vi "Example.vi"() -> ()   [LabVIEW 2014, in "DAQ HVPS.lvclass"]
uses:
  Session Based/DAQ/DAQ HVPS.lvclass
  Session Based/Base/Session HVPS.lvclass
  <userlib>/_Session Fwk/Session - Root.lvclass
  reusable/Session APIs/File Access/Config Data/Config Data.lvclass
  reusable/Session APIs/File Access/Config Data/Config Session.ctl
panel:
  in  "V 2":dbl
  out "x-y":u32
  out "error out":errorcluster
  out "V":dbl
  in  "Boolean":bool
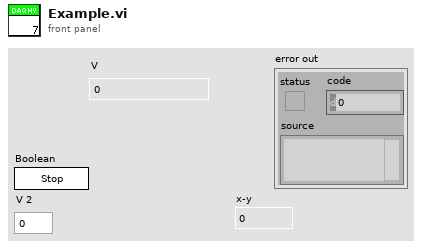
[diagram p1: front panel]
types:
  T1 = typedef "Config Data.lvclass/Config Session.ctl" = refnum<data-value>
  T2 = typedef "Session - Root.lvclass/Session Handle.ctl" = refnum<data-value>
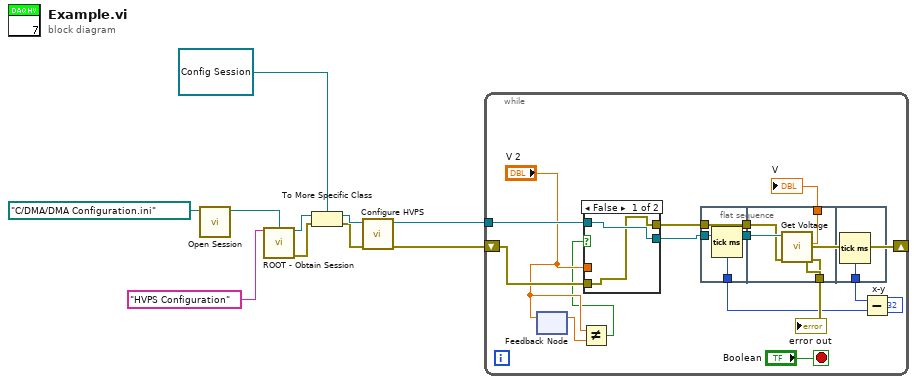
[diagram p0: block diagram]
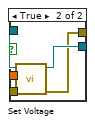
[diagram p2: hidden frame]
diagram:
  n1 = call "Open Session.vi"("Path"=path "C:/DMA/DMA Configuration.ini") -> ("Config Data"=w9:refnum<class "Config Data.lvclass">)  [unwired: 9 in, 1 out]
  n2 = call <userlib>:"ROOT - Obtain Session.vi"("Session Name ()"="HVPS Configuration", "OBJ - Session"=w9) -> ("Session Handle"=w7:T2, "error out"=w3:errorcluster)  [unwired: 11 in, 1 out]
  n3 = To More Specific Class(target class=T1 refnum ("Session Handle"), reference=w7, error in=w3) -> (specific class reference=w5:T1, error out=w4:errorcluster)
  n4 = call "Configure HVPS.vi"("error in"=w4, "Config Handle"=w5) -> ("error out"=w1:errorcluster, "Session HVPS out"=w2:refnum<class "Session HVPS.lvclass">)  [unwired: 8 in]
  n5 = while {
    tunnel: w2 -> [w17]
    shift-right: [w23] -> _
    shift-left: w1 -> [w14]
    stop <- "Boolean" stop-if-true
    n6 = feedback-in #1("V 2") -> ()
    n7 = feedback #1() -> (w13:dbl)  [unwired: 1 in]
    n8 = Not Equal?(x="V 2", y=w13) -> (x != y?=w11:bool)
    n9 = case shown="False" w11 {
      tunnel: w17 -> [w27 w32]
      tunnel: [w27 w31] -> w16
      tunnel: [w26 w30] -> w15
      tunnel: w14 -> [w26 w29]
      tunnel: "V 2" -> [_ w28]
      frame False {
      }
      frame True {
        n10 = call-dynamic "Set Voltage.vi"("error in"=w29, "V"=w28, "Session HVPS in"=w32) -> ("error out"=w30:errorcluster, "Session HVPS out"=w31:refnum<class "Session HVPS.lvclass">)  [unwired: 7 in]
      }
    }
    n11 = flat-sequence {
      tunnel: w15 -> [w34]
      tunnel: w16 -> [w35]
      tunnel: [w35] -> w22
      tunnel: [w34] -> w21
      tunnel: [w33] -> w19
      tunnel: [w37] -> w24
      tunnel: [w36] -> w23
      tunnel: w22 -> [w39]
      tunnel: w21 -> [w38]
      tunnel: [w40] -> w20
      frame #0 {
        n12 = Tick Count (ms)() -> (millisecond timer value=w33:u32)
      }
      frame #1 {
        n13 = call-dynamic "Get Voltage.vi"("error in"=w38, "Session HVPS in"=w39) -> ("error out"=w36:errorcluster, "V"=w37:dbl)  [unwired: 7 in, 1 out]
      }
      frame #2 {
        n14 = Tick Count (ms)() -> (millisecond timer value=w40:u32)
      }
    }
    n15 = Subtract(x=w20, y=w19) -> (x-y=→"x-y":u32)
    "V" <- w24
    "error out" <- w23
  }
